vi "JS Chart.vi"() -> ()   [LabVIEW 2020]
uses:
  Webview2 Control/WebView2 Control.xctl
  Webview2 Lib/WebView2 Control Object/Paths.ctl
  Webview2 Lib/WebView2 Control Object/WebView2 Control.lvclass
panel:
  out "Timed Out":bool
  in  "Chart Label":string
  in  "Stop":bool
  out "Chart":string(xcontrol)
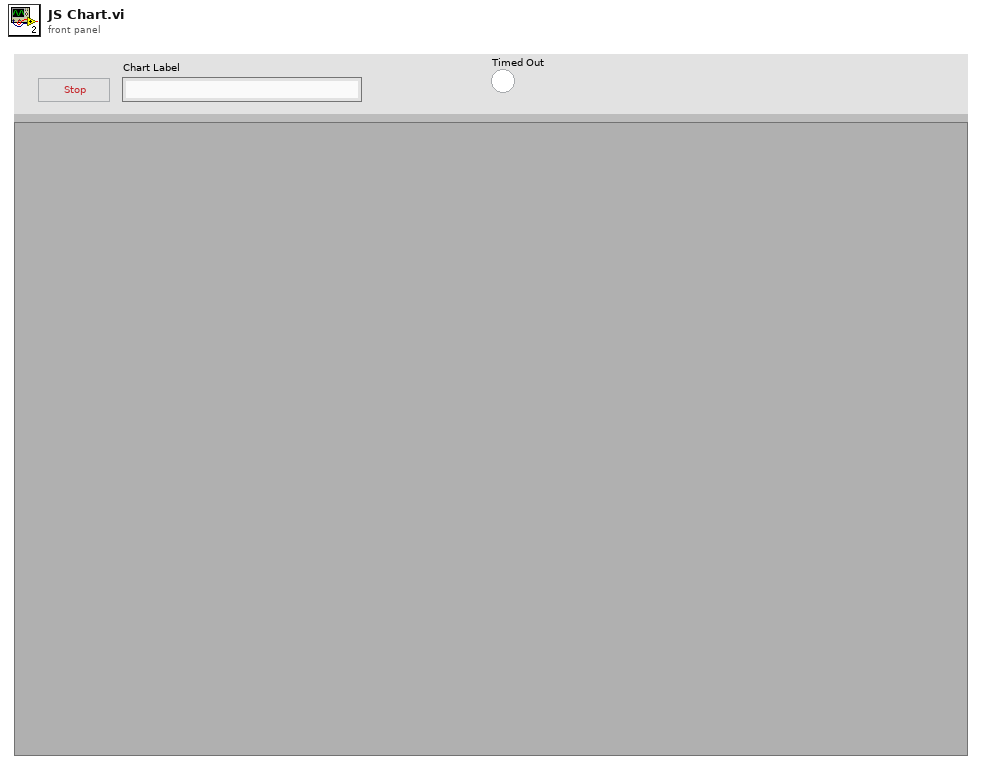
[diagram p1: front panel]
types:
  T1 = typedef "WebView2.lvlib/WebView2 Control.lvclass/Paths.ctl" = cluster{"Webview2 Native":path, "Edge Application":path, "User Data":path}
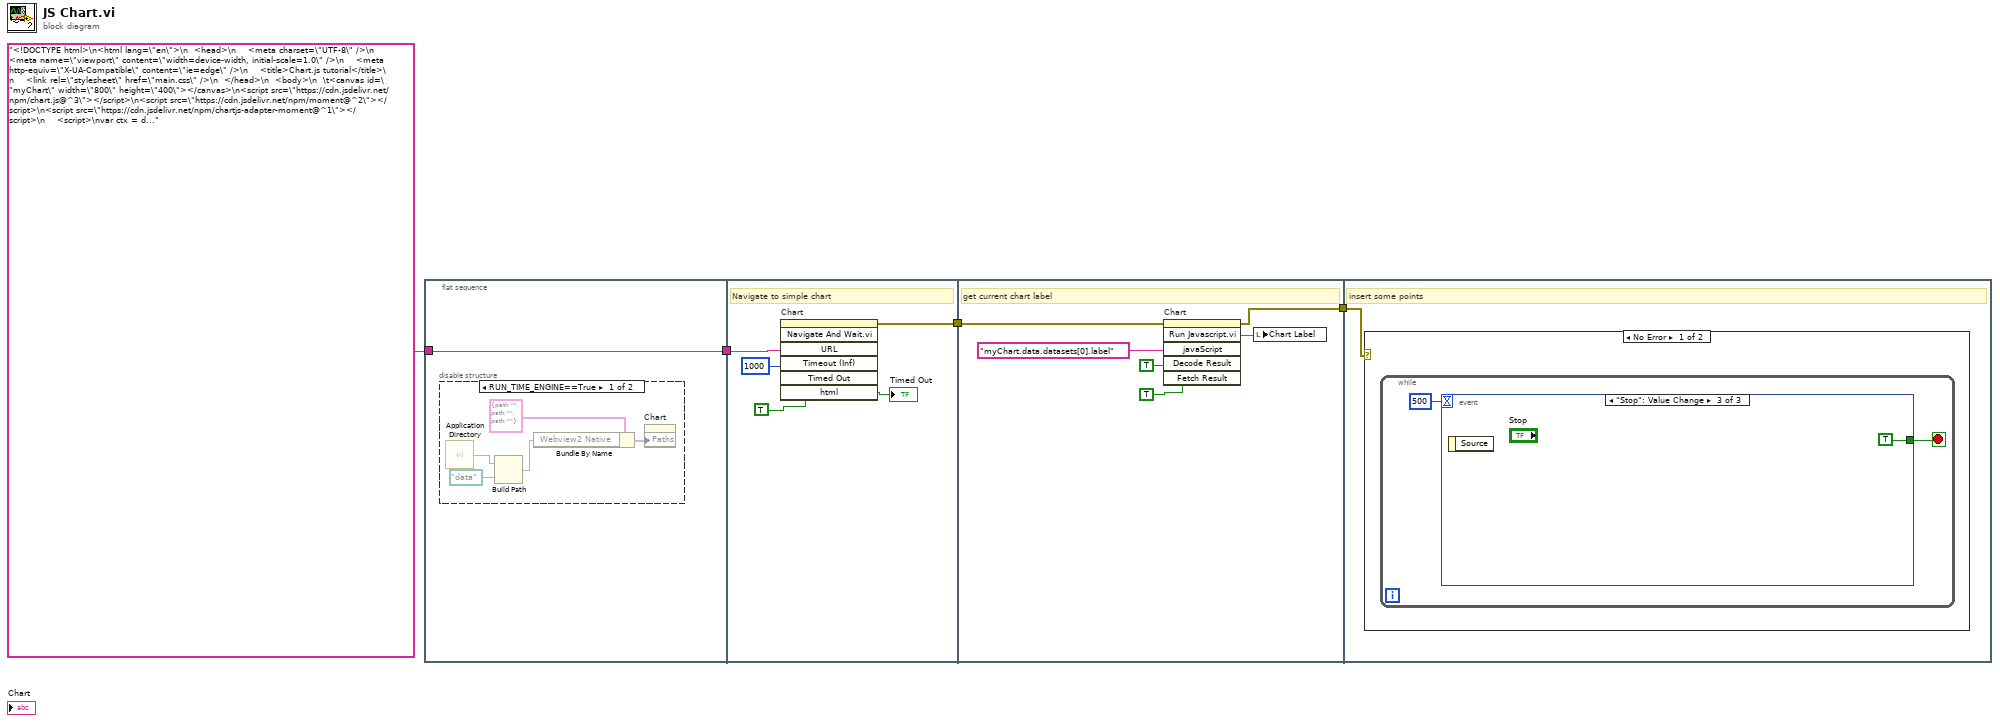
[diagram p0: block diagram]
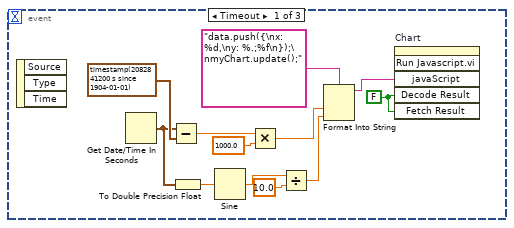
[diagram p3: hidden frame]
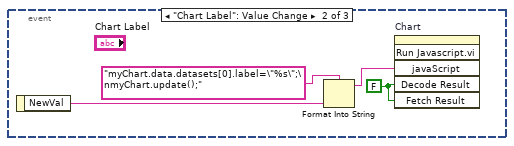
[diagram p4: hidden frame]
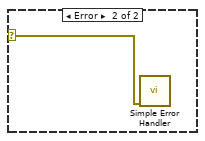
[diagram p5: hidden frame]
diagram:
  n1 = flat-sequence {
    tunnel: "<!DOCTYPE html>\n<html lang=\"en\">\n  <head>\n    <meta charset=\"UTF-8\" />\n    <meta name=\"viewport\" content=\"width=device-width, initial-scale=1.0\" />\n    <meta http-equiv=\"X-UA-Compatible\" content=\"ie=edge\" />\n    <title>Chart.js tutorial</title>\n    <link rel=\"stylesheet\" href=\"main.css\" />\n  </head>\n  <body>\n  \t<canvas id=\"myChart\" width=\"800\" height=\"400\"></canvas>\n<script src=\"https://cdn.jsdelivr.net/npm/chart.js@^3\"></script>\n<script src=\"https://cdn.jsdelivr.net/npm/moment@^2\"></script>\n<script src=\"https://cdn.jsdelivr.net/npm/chartjs-adapter-moment@^1\"></script>\n    <script>\nvar ctx = document.getElementById(\"myChart\");\n\nvar data = []\n\nvar myChart = new Chart(ctx, {\n type: \"line\",\n options: {\n\tscales: {\n\t\tx: {\n\t\t\ttype: 'time'\n\t\t}\n\t}\n },\n data: {\n    datasets: [\n    {\n\t\tlabel: \"Data\",\n        data: data,\n        backgroundColor: \"rgba(255, 99, 132, 0.2)\",\n        borderColor: \"rgba(255, 99, 132, 1)\",\n        borderWidth: 1\n    }\n    ]\n }\n});\n\n\t</script>\n  </body>\n</html>\n" -> [w5]
    tunnel: [w5] -> w1
    tunnel: [w11] -> w2
    tunnel: w1 -> [w12]
    tunnel: [w18] -> w4
    tunnel: w2 -> [w16]
    tunnel: w4 -> [w22]
    frame #0 {
      n2 = disable-structure shown="RUN_TIME_ENGINE==True" {
        frame condition #0 {
          n3 = call <vilib>:"Application Directory.vi"() -> ("Application Directory"=w8:path)
          n4 = Build Path(base path=w8, name or relative path=path "data") -> (appended path=w6:path)
          n5 = Bundle By Name(cluster=T1 {"Webview2 Native"=path "", "Edge Application"=path "", "User Data"=path ""} ("Paths"), "Webview2 Native"=w6) -> (w9:T1)
          n6 = property on="Chart" class="WebView2 Control (strict)"("Paths"=w9) -> ()  [unwired: 2 in, 2 out]
        }
        frame condition #1 (active) {
        }
      }
    }
    frame #1 {
      # "Navigate to simple chart"
      n7 = invoke on="Chart" class="WebView2 Control (strict)" method="Navigate And Wait.vi"("URL"=w12, "Timeout (Inf)"=1000, "html"=TRUE) -> (error out=w11:errorcluster, "Timed Out"=→"Timed Out":bool)  [unwired: 4 in, 5 out]
    }
    frame #2 {
      # "get current chart label"
      n8 = invoke on="Chart" class="WebView2 Control (strict)" method="Run Javascript.vi"(error in=w16, "javaScript"="myChart.data.datasets[0].label", "Decode Result"=TRUE, "Fetch Result"=TRUE) -> (error out=w18:errorcluster, "Run Javascript.vi"=w19:string)  [unwired: 2 in, 4 out]
      n9 = local write "Chart Label"(w19) -> ()
    }
    frame #3 {
      # "insert some points"
      n10 = case shown="No Error" w22 {
        selector: w22 -> [_ w42]
        frame No Error {
          n11 = while {
            stop <- w23 stop-if-true
            n12 = event shown="[2] \"Stop\": Value Change" {
              selector: _ -> [_ _ _]
              dyn-events: _ -> [_ _ _]
              timeout: 500 -> [_ _ _]
              tunnel: [_ _ TRUE] -> w23
              event Timeout {
                w25 = FALSE ("Decode Result")
                n13 = event-data() -> ()  [unwired: 1 in, 3 out]
                n14 = Get Date/Time In Seconds() -> (seconds since 1Jan1904=w27:timestamp)
                n15 = Subtract(x=w27, y=timestamp(2082841200 s since 1904-01-01) ("current time")) -> (x-y=w29:dbl)
                n16 = To Double Precision Float(number=w27) -> (double precision float=w34:dbl)
                n17 = Sine(x=w34) -> (sin(x)=w33:dbl)
                n18 = Multiply(x=w29, y=1000.0) -> (x*y=w26:dbl)
                n19 = Divide(x=w33, y=10.0) -> (x/y=w32:dbl)
                n20 = Format Into String(format string="data.push({\nx: %d,\ny: %.;%f\n});\nmyChart.update();" ("javaScript"), w26, w32) -> (resulting string=w35:string)  [unwired: 2 in, 1 out]
                n21 = invoke on="Chart" class="WebView2 Control (strict)" method="Run Javascript.vi"("javaScript"=w35, "Decode Result"=w25, "Fetch Result"=w25) -> ()  [unwired: 3 in, 6 out]
              }
              event "Chart Label": Value Change {
                w37 = FALSE ("Decode Result")
                n22 = event-data() -> ("NewVal"=w38:string)  [unwired: 1 in]
                n23 = Format Into String(format string="myChart.data.datasets[0].label=\"%s\";\nmyChart.update();" ("javaScript"), w38) -> (resulting string=w39:string)  [unwired: 2 in, 1 out]
                n24 = invoke on="Chart" class="WebView2 Control (strict)" method="Run Javascript.vi"("javaScript"=w39, "Decode Result"=w37, "Fetch Result"=w37) -> ()  [unwired: 3 in, 6 out]
              }
              event "Stop": Value Change {
                n25 = event-data() -> ()  [unwired: 1 in, 1 out]
              }
            }
          }
        }
        frame Error {
          n26 = call <vilib>:"Simple Error Handler.vi"("error in (no error)"=w42) -> ()  [unwired: 4 in, 5 out]
        }
      }
    }
  }
